vi "Maruszak_Pracownia_6.vi"() -> ()   [LabVIEW 2019]
uses:
  Maruszak_Pracownia_6_global.vi
panel:
  in  "stop":bool
  in  "Zero":bool
  out "Liczba binarnie":bool[](array[boolean])
  in  "Liczba":u8
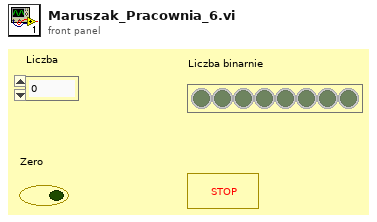
[diagram p1: front panel]
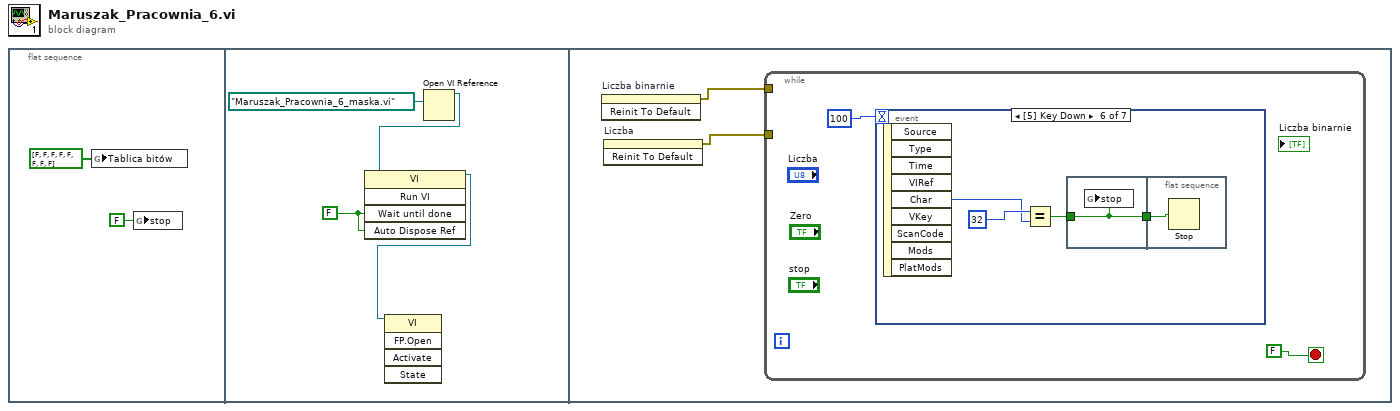
[diagram p0: block diagram]
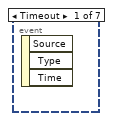
[diagram p2: hidden frame]
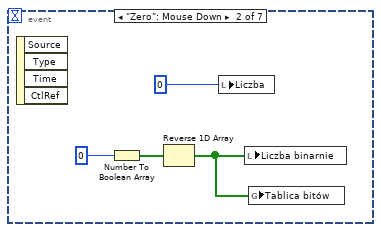
[diagram p3: hidden frame]
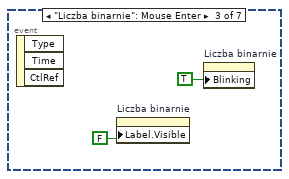
[diagram p4: hidden frame]
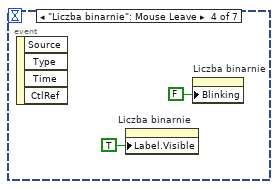
[diagram p5: hidden frame]
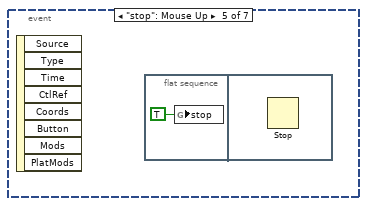
[diagram p6: hidden frame]
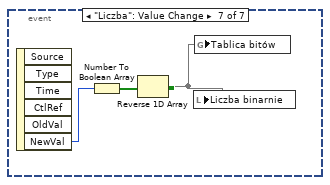
[diagram p7: hidden frame]
diagram:
  n1 = flat-sequence {
    frame #0 {
      n2 = global write "Maruszak_Pracownia_6_global.vi" "Tablica bitów"(bool[] [FALSE, FALSE, FALSE, FALSE, FALSE, FALSE, FALSE, FALSE] ("Tablica bitów")) -> ()
      n3 = global write "Maruszak_Pracownia_6_global.vi" "stop"(FALSE ("stop")) -> ()
    }
    frame #1 {
      w4 = FALSE ("Wait Until Done")
      n4 = Open VI Reference(vi path=path "Maruszak_Pracownia_6_maska.vi") -> (vi reference=w5:refnum<vi>)  [unwired: 5 in, 1 out]
      n5 = invoke class="VI" method="Run VI"(reference=w5, "Wait until done"=w4, "Auto Dispose Ref"=w4) -> (reference out=w3:refnum<vi>)  [unwired: 2 in, 4 out]
      n6 = invoke class="VI" method="FP.Open"(reference=w3) -> ()  [unwired: 4 in, 5 out]
    }
    frame #2 {
      n7 = invoke on="Liczba binarnie" class="Arr (strict)" method="Reinit To Default"() -> (error out=w7:errorcluster)  [unwired: 3 in, 2 out]
      n8 = invoke on="Liczba" class="DigNum (strict)" method="Reinit To Default"() -> (error out=w8:errorcluster)  [unwired: 3 in, 2 out]
      n9 = while {
        tunnel: w8 -> [_]
        tunnel: w7 -> [_]
        stop <- FALSE stop-if-true
        n10 = event shown="[5] Key Down" {
          selector: _ -> [_ _ _ _ _ _ _]
          dyn-events: _ -> [_ _ _ _ _ _ _]
          timeout: 100 -> [_ _ _ _ _ _ _]
          event Timeout {
            n11 = event-data() -> ()  [unwired: 1 in, 3 out]
          }
          event "Zero": Mouse Down {
            n12 = event-data() -> ()  [unwired: 1 in, 4 out]
            n13 = Number To Boolean Array(number=u8 0) -> (Boolean array=w12:bool[])
            n14 = Reverse 1D Array(array=w12) -> (reversed array=w11:bool[])
            n15 = local write "Liczba"(u8 0 ("Liczba")) -> ()
            n16 = local write "Liczba binarnie"(w11) -> ()
            n17 = global write "Maruszak_Pracownia_6_global.vi" "Tablica bitów"(w11) -> ()
          }
          event "Liczba binarnie": Mouse Enter {
            n18 = event-data() -> ()  [unwired: 1 in, 3 out]
            n19 = property on="Liczba binarnie" class="Arr (strict)"("Label.Visible"=FALSE) -> ()  [unwired: 2 in, 2 out]
            n20 = property on="Liczba binarnie" class="Arr (strict)"("Blinking"=TRUE) -> ()  [unwired: 2 in, 2 out]
          }
          event "Liczba binarnie": Mouse Leave {
            n21 = event-data() -> ()  [unwired: 1 in, 4 out]
            n22 = property on="Liczba binarnie" class="Arr (strict)"("Label.Visible"=TRUE) -> ()  [unwired: 2 in, 2 out]
            n23 = property on="Liczba binarnie" class="Arr (strict)"("Blinking"=FALSE) -> ()  [unwired: 2 in, 2 out]
          }
          event "stop": Mouse Up {
            n24 = event-data() -> ()  [unwired: 1 in, 8 out]
            n25 = flat-sequence {
              frame #0 {
                n26 = global write "Maruszak_Pracownia_6_global.vi" "stop"(TRUE ("stop")) -> ()
              }
              frame #1 {
                n27 = Stop() -> ()  [unwired: 1 in]
              }
            }
          }
          event Key Down {
            n28 = event-data() -> ("Char"=w22:i16)  [unwired: 1 in, 8 out]
            n29 = Equal?(x=i16 32, y=w22) -> (x = y?=w21:bool)
            n30 = flat-sequence {
              tunnel: w21 -> [w24]
              tunnel: [w24] -> w20
              tunnel: w20 -> [w25]
              frame #0 {
                n31 = global write "Maruszak_Pracownia_6_global.vi" "stop"(w24) -> ()
              }
              frame #1 {
                n32 = Stop(stop? (T)=w25) -> ()
              }
            }
          }
          event "Liczba": Value Change {
            n33 = event-data() -> ("NewVal"=w28:u8)  [unwired: 1 in, 5 out]
            n34 = Number To Boolean Array(number=w28) -> (Boolean array=w27:bool[])
            n35 = Reverse 1D Array(array=w27) -> (reversed array=w26:bool[])
            n36 = local write "Liczba binarnie"(w26) -> ()
            n37 = global write "Maruszak_Pracownia_6_global.vi" "Tablica bitów"(w26) -> ()
          }
        }
      }
    }
  }
